vi "create_pipettes.vi"   [LabVIEW 2015]
doc: "reads the Pipettes.ini and creates the pipette objects"
uses:
  Classes/Pipette/Pipette.lvclass
  <vilib>/Utility/config.llb/Read Key (Double).vi
  <vilib>/Utility/config.llb/Read Key (String).vi
  <vilib>/Utility/config.llb/Read Key (U32).vi
  <vilib>/Utility/config.llb/NI_LVConfig.lvlib
types:
  T1 = typedef "NI_LVConfig.lvlib/Config Data RefNum.ctl" = refnum<k1>
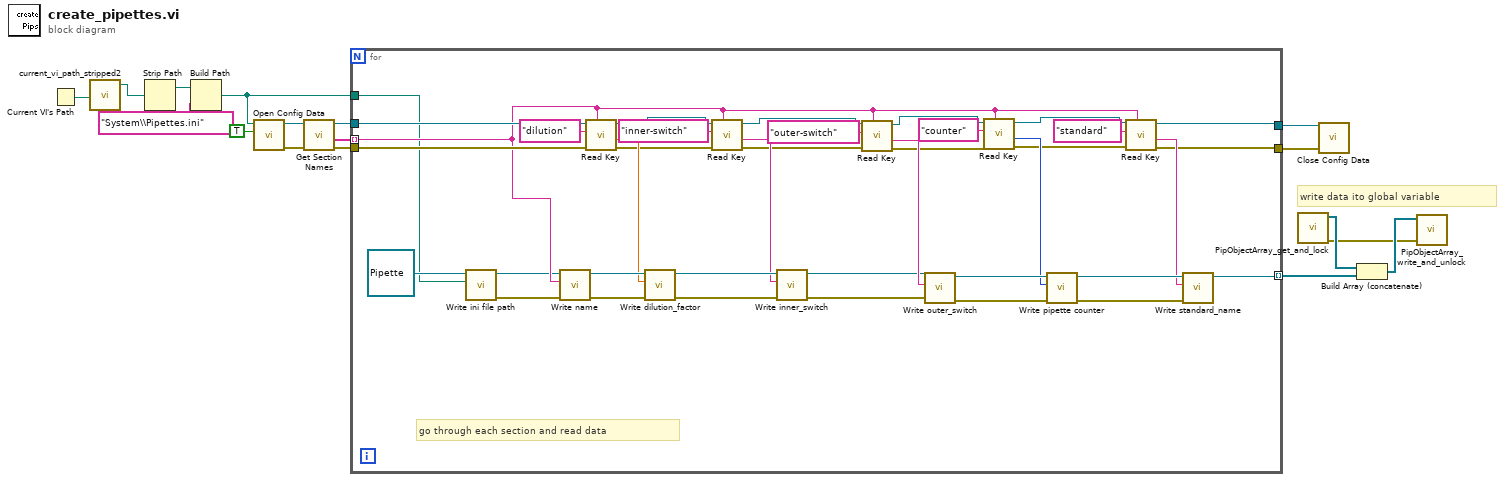
[diagram p0: block diagram]
diagram:
  # "write data ito global variable"
  n1 = Current VI's Path() -> (path=w12:path)
  n2 = call "current_vi_path_stripped2.vi"("current VI Path"=w12) -> ("current VI Path stripped out"=w8:path)  [unwired: 3 in, 1 out]
  n3 = Strip Path(path=w8) -> (stripped path=w9:path)  [unwired: 1 out]
  n4 = Build Path(base path=w9, name or relative path="System\\Pipettes.ini") -> (appended path=w1:path)
  n5 = call <vilib>:"Open Config Data.vi"("create file if necessary (T)"=TRUE, "configuration file path"=w1) -> ("error out"=w13:errorcluster, "refnum"=w14:T1)  [unwired: 7 in, 1 out]
  n6 = call <vilib>:"Get Section Names.vi"("error in (no error)"=w13, "refnum"=w14) -> ("error out"=w17:errorcluster, "section names"=w15:string[], "refnum out"=w16:T1)  [unwired: 7 in]
  n7 = for {
    tunnel: w15 -> [w30] mode=indexing
    tunnel: w16 -> [w52]
    tunnel: w17 -> [w51]
    tunnel: [w24] -> w4 mode=indexing
    tunnel: [w23] -> w7
    tunnel: [w22] -> w6
    tunnel: w1 -> [w18]
    # "go through each section and read data"
    n8 = call-dynamic "Write ini file path.vi"("ini file path"=w18, "Pipette in"=refnum<class "Pipette.lvclass"> refnum ("Pipette.lvclass")) -> ("error out"=w19:errorcluster, "Pipette out"=w20:refnum<class "Pipette.lvclass">)  [unwired: 8 in]
    n9 = call-dynamic "Write name.vi"("error in (no error)"=w19, "name"=w30, "Pipette in"=w20) -> ("error out"=w54:errorcluster, "Pipette out"=w55:refnum<class "Pipette.lvclass">)  [unwired: 7 in]
    n10 = call-poly <vilib>:"Read Key.vi"("section"=w30, "error in (no error)"=w51, "key"="dilution", "refnum"=w52) -> ("error out"=w47:errorcluster, "value"=w50:dbl, "refnum out"=w48:T1)  [unwired: 4 in, 1 out]
    n11 = call-dynamic "Write dilution_factor.vi"("error in (no error)"=w54, "dilution_factor"=w50, "Pipette in"=w55) -> ("error out"=w45:errorcluster, "Pipette out"=w46:refnum<class "Pipette.lvclass">)  [unwired: 7 in]
    n12 = call-poly <vilib>:"Read Key.vi"("section"=w30, "error in (no error)"=w47, "key"="inner-switch", "refnum"=w48) -> ("error out"=w41:errorcluster, "value"=w44:string, "refnum out"=w42:T1)  [unwired: 4 in, 1 out]
    n13 = call-dynamic "Write inner_switch.vi"("error in (no error)"=w45, "inner_switch"=w44, "Pipette in"=w46) -> ("error out"=w38:errorcluster, "Pipette out"=w39:refnum<class "Pipette.lvclass">)  [unwired: 7 in]
    n14 = call-poly <vilib>:"Read Key.vi"("section"=w30, "error in (no error)"=w41, "key"="outer-switch", "refnum"=w42) -> ("error out"=w35:errorcluster, "value"=w40:string, "refnum out"=w36:T1)  [unwired: 4 in, 1 out]
    n15 = call-dynamic "Write outer_switch.vi"("error in (no error)"=w38, "outer_switch"=w40, "Pipette in"=w39) -> ("error out"=w33:errorcluster, "Pipette out"=w34:refnum<class "Pipette.lvclass">)  [unwired: 7 in]
    n16 = call-poly <vilib>:"Read Key.vi"("section"=w30, "error in (no error)"=w35, "key"="counter", "refnum"=w36) -> ("error out"=w28:errorcluster, "value"=w32:u32, "refnum out"=w29:T1)  [unwired: 4 in, 1 out]
    n17 = call-dynamic "Write pipette counter.vi"("error in (no error)"=w33, "pipette counter"=w32, "Pipette in"=w34) -> ("error out"=w26:errorcluster, "Pipette out"=w27:refnum<class "Pipette.lvclass">)  [unwired: 7 in]
    n18 = call-poly <vilib>:"Read Key.vi"("section"=w30, "error in (no error)"=w28, "key"="standard", "refnum"=w29) -> ("error out"=w22:errorcluster, "value"=w25:string, "refnum out"=w23:T1)  [unwired: 4 in, 1 out]
    n19 = call-dynamic "Write standard_name.vi"("error in (no error)"=w26, "standard_name"=w25, "Pipette in"=w27) -> ("Pipette out"=w24:refnum<class "Pipette.lvclass">)  [unwired: 7 in, 1 out]
  }
  n20 = call "PipObjectArray_get_and_lock.vi"() -> ("error out"=w2:errorcluster, "PipObjects"=w5:refnum<class "Pipette.lvclass">[])  [unwired: 10 in]
  n21 = call <vilib>:"Close Config Data.vi"("error in (no error)"=w6, "refnum"=w7) -> ()  [unwired: 8 in, 2 out]
  n22 = Build Array (concatenate)(w5, w4) -> (w3:refnum<class "Pipette.lvclass">[])
  n23 = call "PipObjectArray_write_and_unlock.vi"("error in (no error)"=w2, "PipObjects"=w3) -> ()  [unwired: 9 in, 1 out]
